vi "Insert Brower Panel in Subpanel.vi"(8 "error in (no error)":errorcluster, 10 "Brower Subpanel Refnum":refnum<vi>, 11 "Browers in":refnum<class "Browers Controller.lvclass">) -> (0 "error out":errorcluster, 3 "Browers out":refnum<class "Browers Controller.lvclass">)   [LabVIEW 2015, in "Browers Controller.lvclass"]
uses:
  Browers Controller.lvclass
  Browers Controller.lvclass/Browers Controller.ctl
  Brower View/Brower View.lvclass/Brower View.ctl
  Brower View/Brower View.lvclass
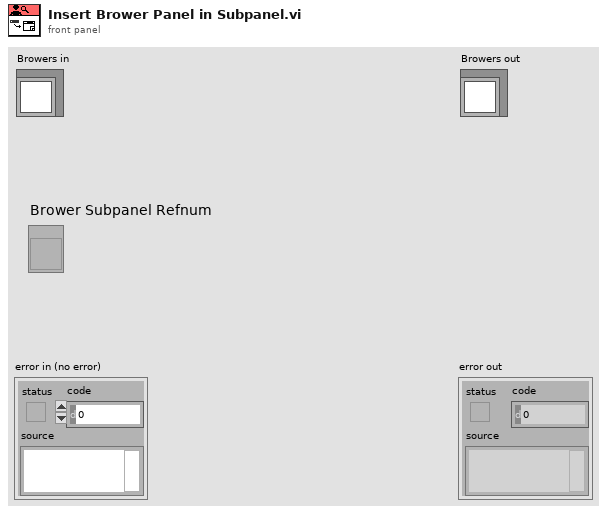
[diagram p1: front panel]
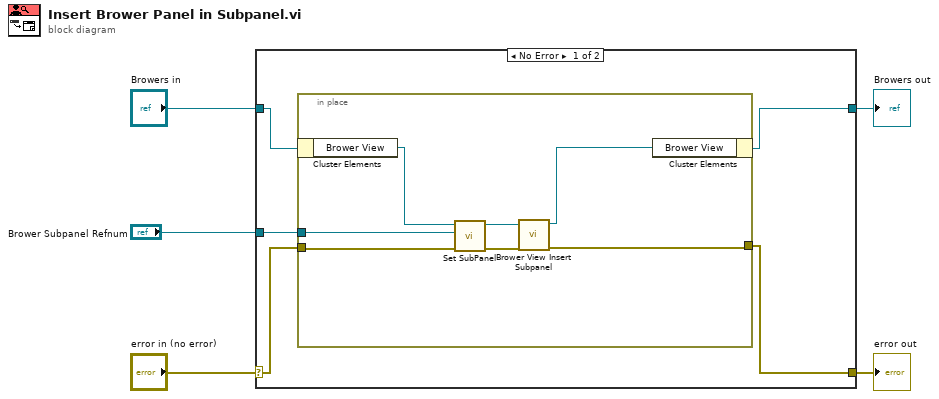
[diagram p0: block diagram]
diagram:
  n1 = case shown="No Error" "error in (no error)" {
    selector: "error in (no error)" -> [w9 w19]
    tunnel: [w7 w19] -> w4
    tunnel: [w6 w18] -> w2
    tunnel: "Browers in" -> [w8 w18]
    tunnel: "Brower Subpanel Refnum" -> [w10 _]
    frame No Error {
      n2 = in-place {
        in-place-border: w10 -> [w17]
        in-place-border: w9 -> [w16]
        in-place-border: [w11] -> w7
        n3 = in-place-cluster #1(w8) -> ("Brower View"=w13:refnum<class "Brower View.lvclass">)
        n4 = call "Set SubPanel.vi"("error in (no error)"=w16, "SubPanel"=w17, "Brower View in"=w13) -> ("error out"=w14:errorcluster, "Brower View out"=w15:refnum<class "Brower View.lvclass">)  [unwired: 7 in]
        n5 = call "Brower View Insert Subpanel.vi"("error in (no error)"=w14, "Brower View in"=w15) -> ("error out"=w11:errorcluster, "Brower View out"=w12:refnum<class "Brower View.lvclass">)  [unwired: 8 in]
        n6 = in-place-cluster #1("Brower View"=w12) -> (w6:refnum<class "Browers Controller.lvclass">)
      }
    }
    frame Error {
    }
  }
  "error out" <- w4
  "Browers out" <- w2
